vi "Querry.vi"(8 "error in (no error)":errorcluster, 10 "PDU_req":T1={"Function Code"=1, "Data"=[], "RTU_DataBytes"=0}, 11 "MB_Serial session in":refnum<class "MB_Master_Serial.lvclass">) -> (0 "error out":errorcluster, 2 "PDU_resp":T1={"Function Code"=1, "Data"=[], "RTU_DataBytes"=0}, 3 "MB_Serial session out":refnum<class "MB_Master_Serial.lvclass">)   [LabVIEW 2016, in "MB Master.lvlib" / "MB_Master_Serial.lvclass"]
doc: "Transmits the PDU request and receives the PDU response as an atomic operation. The session is reserved by a mutex and the com port is reserved using VISA lock."
uses:
  MB_Master_Serial.lvclass
  MB_PDU/MB_PDU_Cluster.ctl
  MB_Master_Serial.lvclass/MB_Master_Serial.ctl
  MB_ADU_TCP/MB_ADU_Serial/MB_ADU_Serial.lvclass
  MB_VISA_Lock/MB_VISA_Lock.lvlib
  MB Master.lvlib
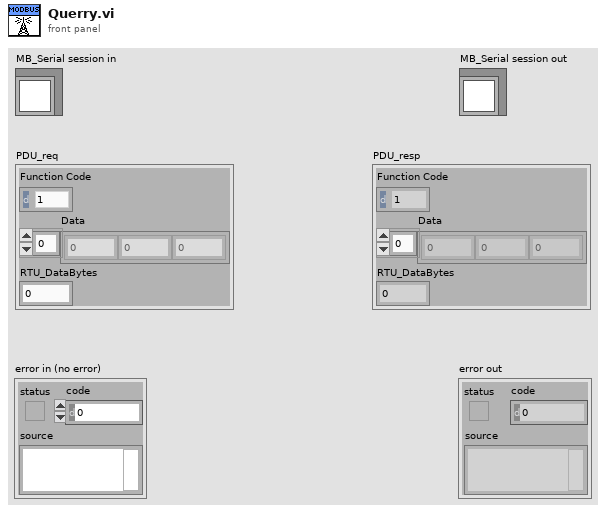
[diagram p1: front panel]
types:
  T1 = typedef "MB Master.lvlib/MB_PDU_Cluster.ctl" = cluster{"Function Code":u8, "Data":u8[], "RTU_DataBytes":i32}
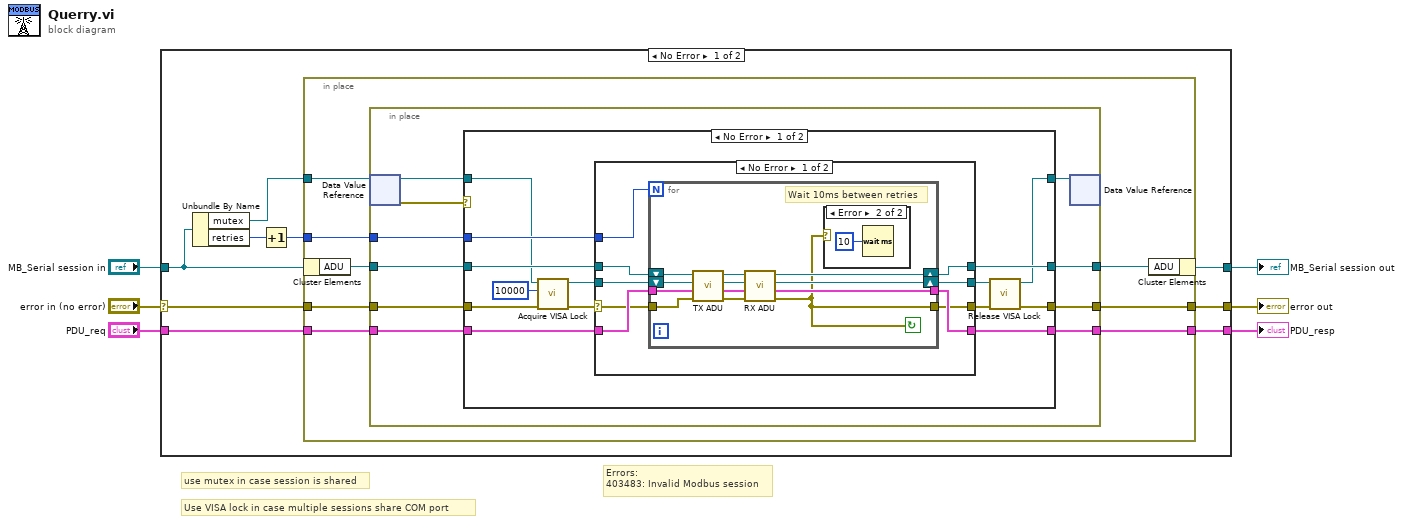
[diagram p0: block diagram]
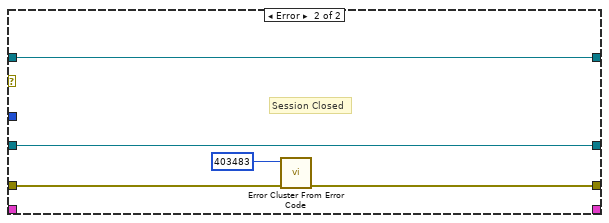
[diagram p4: hidden frame]
diagram:
  # "use mutex in case session is shared"
  # "Use VISA lock in case multiple sessions share COM port"
  # "Errors:\n403483: Invalid Modbus session"
  n1 = case shown="No Error" "error in (no error)" {
    selector: "error in (no error)" -> [w15 w79]
    tunnel: [w14 w79] -> w5
    tunnel: [w12 w78] -> w3
    tunnel: "MB_Serial session in" -> [w13 w78]
    tunnel: "PDU_req" -> [w11 _]
    tunnel: [w10 _] -> w1
    frame No Error {
      n2 = Unbundle By Name(w13) -> ("mutex"=w9:refnum<data-value>, "retries"=w8:i32)
      n3 = Increment(x=w8) -> (x+1=w7:i32)
      n4 = in-place {
        in-place-border: w15 -> [w23]
        in-place-border: [w22] -> w14
        in-place-border: w7 -> [w21]
        in-place-border: w11 -> [w18]
        in-place-border: [w17] -> w10
        in-place-border: w9 -> [w20]
        n5 = in-place-cluster #1(w13) -> ("ADU"=w19:refnum<class "MB_ADU_Serial.lvclass">)
        n6 = in-place {
          in-place-border: w23 -> [w33]
          in-place-border: [w32] -> w22
          in-place-border: w21 -> [w31]
          in-place-border: w19 -> [w30]
          in-place-border: [w29] -> w16
          in-place-border: w18 -> [w27]
          in-place-border: [w26] -> w17
          n7 = in-place-dvr #2(w20) -> (w25:refnum<visa-resource-name>, w28:errorcluster)
          n8 = case shown="No Error" w28 {
            tunnel: w33 -> [w42 w75]
            tunnel: [w38 w74] -> w32
            tunnel: w31 -> [w46 _]
            tunnel: w30 -> [w45 w77]
            tunnel: [w36 w73] -> w24
            tunnel: [w47 w77] -> w29
            tunnel: w27 -> [w44 _]
            tunnel: [w43 _] -> w26
            tunnel: w25 -> [w40 w73]
            frame No Error {
              n9 = call "Acquire VISA Lock.vi"("error in (no error)"=w42, "timeout in ms (-1)"=10000, "VISA resource name"=w40) -> ("error out"=w35:errorcluster, "VISA resource name out"=w41:refnum<visa-resource-name>)  [unwired: 7 in]
              n10 = case shown="No Error" w35 {
                selector: w35 -> [w48 w72]
                tunnel: [w56 w70] -> w47
                tunnel: w46 -> [w55 _]
                tunnel: w45 -> [w54 w70]
                tunnel: w44 -> [w53 _]
                tunnel: [w52 _] -> w43
                tunnel: w41 -> [w51 w71]
                tunnel: [w50 w72] -> w39
                tunnel: [w49 w71] -> w37
                frame No Error {
                  n11 = for {
                    N: w55 -> [_]
                    shift-right: [w62] -> w56
                    shift-left: w54 -> [w68]
                    shift-right: [w61] -> w49
                    shift-left: w51 -> [w66]
                    tunnel: w48 -> [w67]
                    tunnel: [w57] -> w50
                    tunnel: w53 -> [w60]
                    tunnel: [w58] -> w52
                    stop <- w57 continue-if-true
                    # "Wait 10ms between retries"
                    n12 = call-dynamic "TX ADU.vi"("error in (no error)"=w67, "PDU_req in"=w60, "VISA resource in"=w66, "MB_ADU in"=w68) -> ("error out"=w64:errorcluster, "PDU_req out"=w59:T1, "VISA resource out"=w63:refnum<visa-resource-name>, "MB_ADU out"=w65:refnum<class "MB_ADU_Serial.lvclass">)  [unwired: 4 in]
                    n13 = call-dynamic "RX ADU.vi"("error in (no error)"=w64, "PDU_req"=w59, "VISA resource in"=w63, "MB_ADU in"=w65) -> ("error out"=w57:errorcluster, "PDU_resp"=w58:T1, "VISA resource out"=w61:refnum<visa-resource-name>, "MB_ADU out"=w62:refnum<class "MB_ADU_Serial.lvclass">)  [unwired: 4 in]
                    n14 = case shown="Error" w57 {
                      frame No Error {
                      }
                      frame Error {
                        n15 = Wait (ms)(milliseconds to wait=u32 10) -> ()  [unwired: 1 out]
                      }
                    }
                  }
                }
                frame Error {
                  # "Failed to acquire VISA resource lock"
                }
              }
              n16 = call "Release VISA Lock.vi"("error in (no error)"=w39, "VISA resource name"=w37) -> ("error out"=w38:errorcluster, "VISA resource name out"=w36:refnum<visa-resource-name>)  [unwired: 8 in]
            }
            frame Error {
              # "Session Closed"
              n17 = call <vilib>:"Error Cluster From Error Code.vi"("error in (no error)"=w75, "error code (0)"=403483) -> ("error out"=w74:errorcluster)  [unwired: 7 in]
            }
          }
          n18 = in-place-dvr #2(w24) -> ()  [unwired: 2 out]
        }
        n19 = in-place-cluster #1("ADU"=w16) -> (w12:refnum<class "MB_Master_Serial.lvclass">)
      }
    }
    frame Error {
    }
  }
  "error out" <- w5
  "MB_Serial session out" <- w3
  "PDU_resp" <- w1
